vi "DAQ-Hybrid Engine.vi"() -> ()   [LabVIEW 2013]
uses:
  <vilib>/DAQmx/read.llb/DAQmx Read (Analog 1D DBL NChan 1Samp).vi
  <vilib>/Analysis/baseanly.llb/Mean (DBL).vi
  <vilib>/DAQmx/create/channels.llb/DAQmx Create Channel (AI-Voltage-Basic).vi
  <vilib>/DAQmx/configure/timing.llb/DAQmx Timing (Sample Clock).vi
  <vilib>/DAQmx/configure/task.llb/DAQmx Configure Logging (TDMS).vi
  <vilib>/DAQmx/miscellaneous.llb/DAQmx Fill In Error Info.vi
  <resource>/objmgr/daqmx.rc
  <vilib>/Analysis/NI_AALBase.lvlib
panel:
  out "Numeric 2":dbl
  out "Thermometer":dbl(slide) scale=0.0..100.0
  out "Numeric":dbl
  out "Waveform Chart":waveform(dbl)(graph)
  out "?":dbl
  out "Raw":dbl
  in  "File Path 2":path=path "test1.tdms"
  in  "Thrust Offset":dbl format="%0.2f"
  in  "Thrust Slope":dbl=1.0 format="%0.4f"
  in  "Pressure 1 Offset":dbl format="%0.4f"
  in  "Pressure 1 Slope":dbl=1.0 format="%0.2f"
  out "?":dbl
  out "Thrust":dbl(slide) scale=-350.0..350.0
  out "?":dbl
  out "Pressure 1":dbl(knob) scale=0.0..2000.0
  in  "Pressure 1":tag
  in  "?":bool
  in  "?":string="Job 1 - Day 1"
  in  "?":bool
  out "Number of Sensors":sgl
  in  "?":bool
  in  "Samples Per Update":dbl=100.0
  out "Current Group":string="Group 0"
  in  "Sampling Rate [Hz]":i32=10000
  in  "Logging Mode":i32(ring)=15842 items=["Off"=10231, "Log"=15844, "Log and Read"=15842]
  in  "File Path":path=path "test1.tdms"
  # "Data Logging Settings"
  # "Sensor Settings"
  # "Sampling Settings"
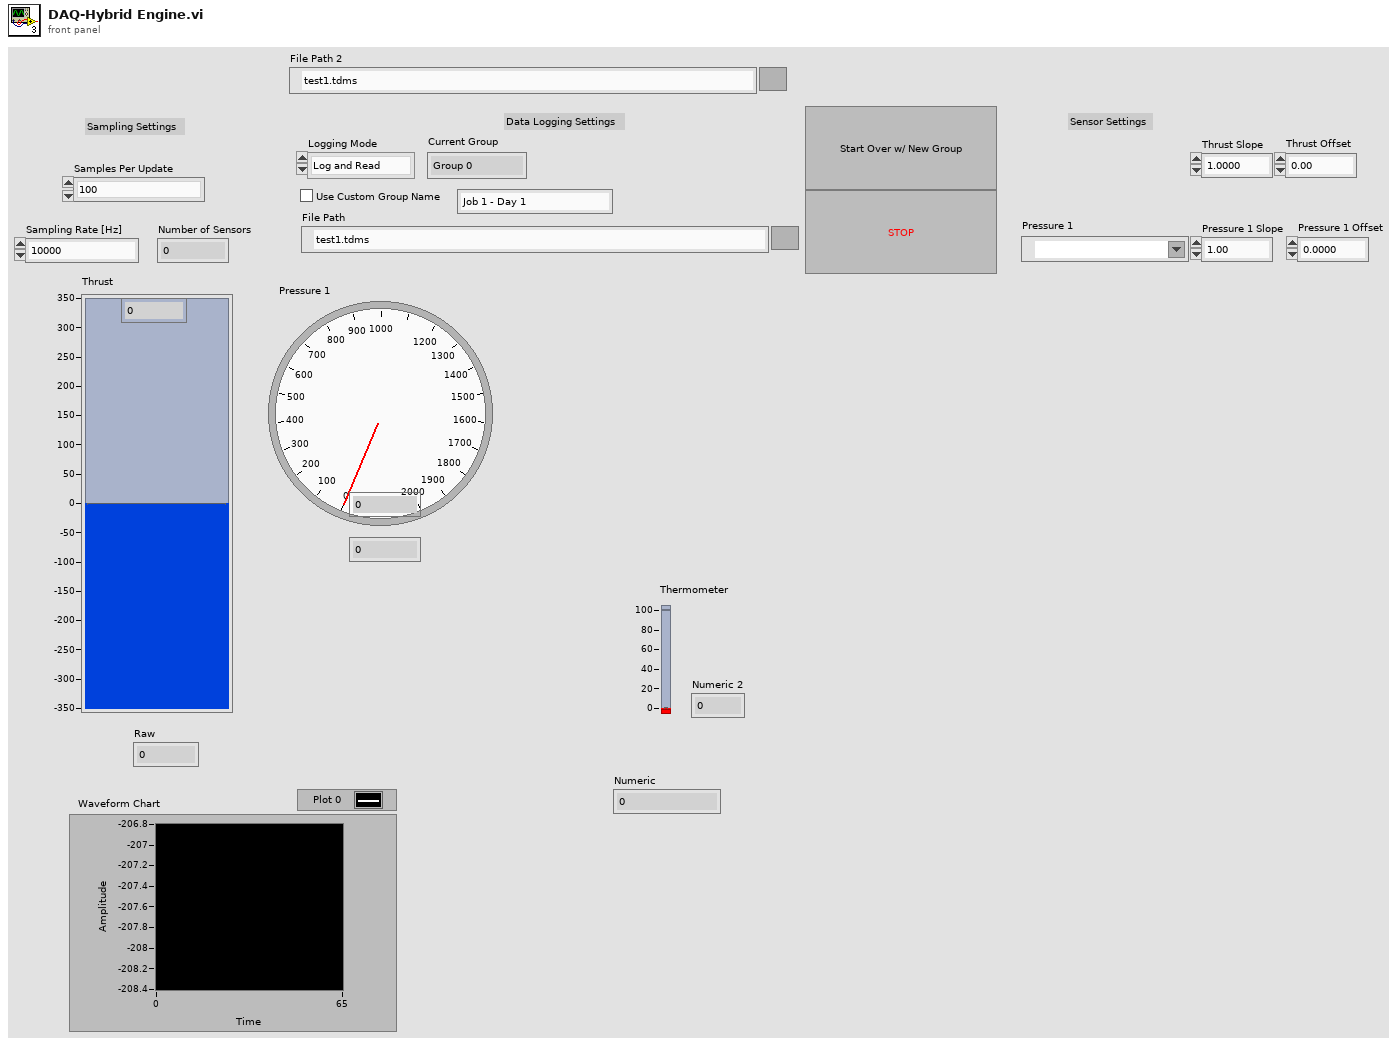
[diagram p1: front panel]
types:
  T1 = enum16{"open", "open or create", "create or replace", "create", "open (read-only)"}
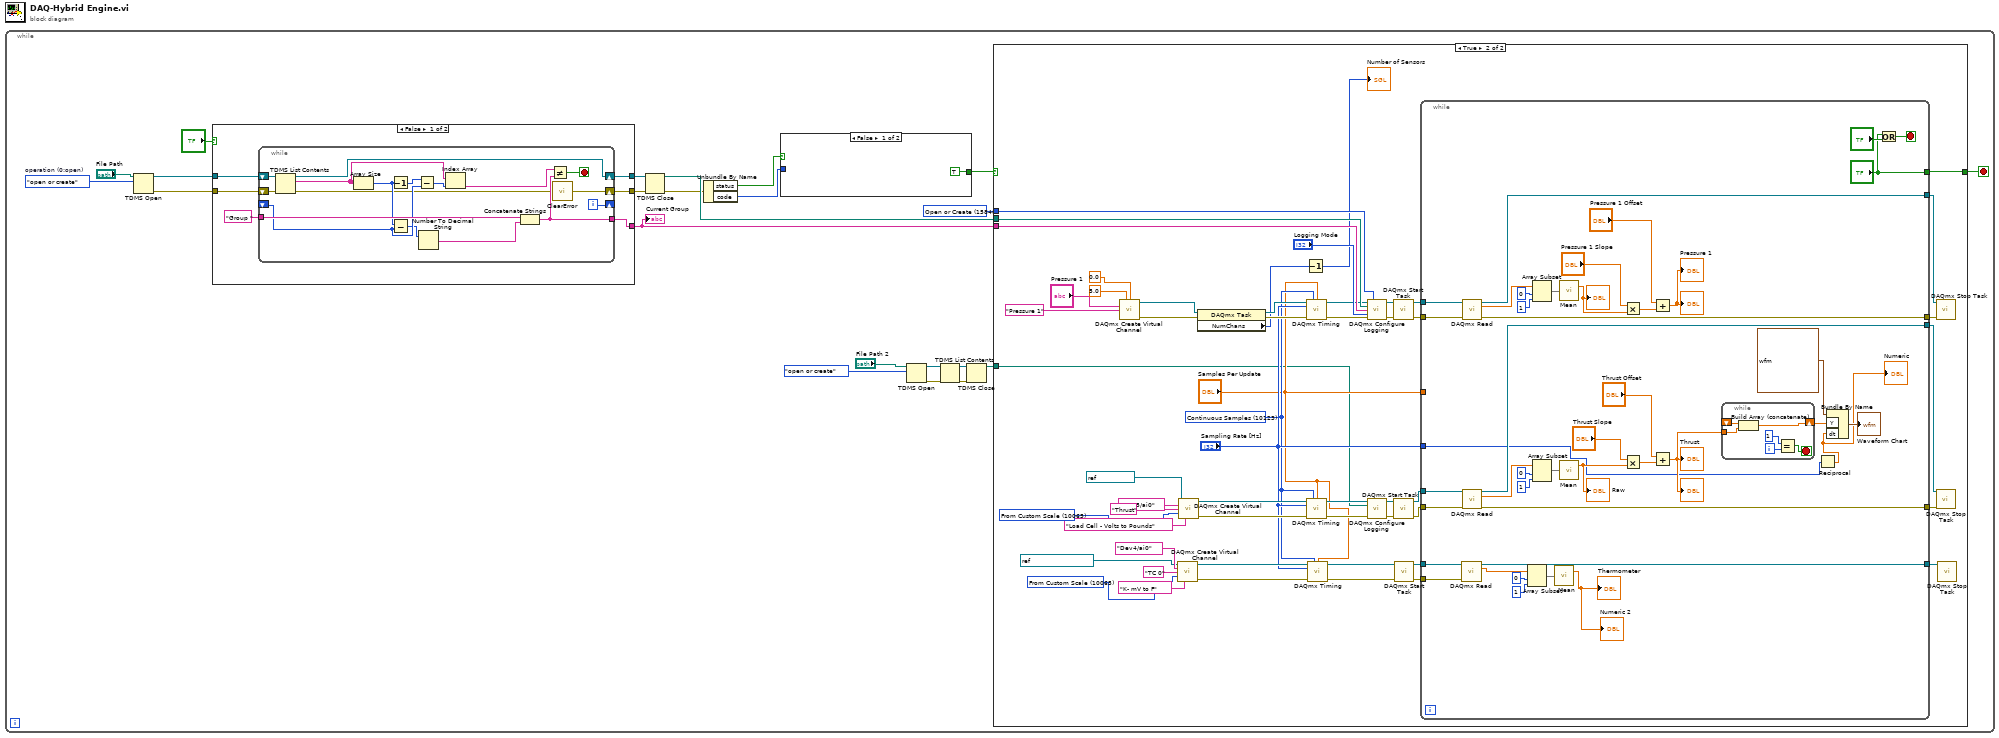
[diagram p0: block diagram]
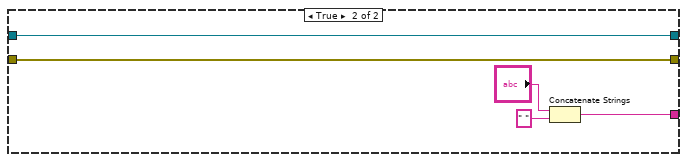
[diagram p2: hidden frame]
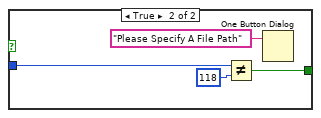
[diagram p3: hidden frame]
diagram:
  n1 = while {
    stop <- w13 stop-if-true
    w19 = T1."open or create"  # operation (0:open)
    w22 = 15846 items=["Open"=10437, "Open or Create"=15846, "Create or Replace"=15847, "Create"=15848] ("operation")
    n2 = TDMS Open(10:w19, 11:"File Path") -> (0:w11:errorcluster, 3:w12:refnum<k34>)  [unwired: 5 in]
    n3 = case shown="False" "?" {
      tunnel: [w25 w48] -> w8
      tunnel: w12 -> [w28 w47]
      tunnel: w11 -> [w27 w46]
      tunnel: [w24 w47] -> w10
      tunnel: [w23 w46] -> w9
      frame False {
        n4 = while {
          shift-right: [w44] -> w24
          shift-left: w28 -> [w45]
          shift-right: [w42] -> w23
          shift-left: w27 -> [w43]
          tunnel: "Group " -> [w40]
          tunnel: [w37] -> w25
          shift-right: [w33] -> _
          shift-left: _ -> [w31]
          i -> [w33]
          stop <- w38 stop-if-true
          n5 = TDMS List Contents(4:w43, 7:w45) -> (0:w29:errorcluster, 2:w36:string[], 3:w44:refnum<k34>)  [unwired: 1 in, 1 out]
          n6 = Array Size(array=w36) -> (size(s)=w32:i32)
          n7 = Decrement(x=w32) -> (x-1=w34:i32)
          n8 = Subtract(x=w32, y=w31) -> (x-y=w30:i32)
          n9 = Subtract(x=w34, y=w31) -> (x-y=w35:i32)
          n10 = Number To Decimal String(number=w30) -> (decimal integer string=w41:string)  [unwired: 1 in]
          n11 = Index Array "Index Array"(array=w36, index=w35) -> (element=w39:string)
          n12 = Concatenate Strings(w40, w41) -> (w37:string)
          n13 = Not Equal?(x=w39, y=w37) -> (x != y?=w38:bool)
          n14 = call <vilib>:"ClearError.vi"("error in (no error)"=w29) -> ("error out"=w42:errorcluster)
        }
      }
      frame True {
        n15 = Concatenate Strings "Concatenate Strings"("?", " ") -> (w48:string)
      }
    }
    "Current Group" <- w8
    n16 = TDMS Close(8:w9, 11:w10) -> (0:w18:errorcluster, 3:w20:path)
    n17 = Unbundle By Name "Unbundle By Name"(w18) -> ("status"=w17:bool, "code"=w16:i32)
    n18 = case shown="False" w17 {
      tunnel: w16 -> [_ w54]
      tunnel: [TRUE w53] -> w15
      frame False {
      }
      frame True {
        n19 = Not Equal?(x=w54, y=118) -> (x != y?=w53:bool)
        n20 = One Button Dialog(message="Please Specify A File Path") -> ()  [unwired: 1 in, 1 out]
      }
    }
    n21 = TDMS Open(10:T1."open or create" ("operation (0:open)"), 11:"File Path 2") -> (0:w4:errorcluster, 3:w5:refnum<k34>)  [unwired: 5 in]
    n22 = TDMS List Contents(4:w4, 7:w5) -> (0:w2:errorcluster, 3:w3:refnum<k34>)  [unwired: 1 in, 2 out]
    n23 = TDMS Close(8:w2, 11:w3) -> (3:w1:path)  [unwired: 1 out]
    n24 = case shown="True" w15 {
      selector: w15 -> [w56 _]
      tunnel: w22 -> [_ w106]
      tunnel: w20 -> [_ w105]
      tunnel: w8 -> [_ w104]
      tunnel: [w56 w95] -> w13
      tunnel: w1 -> [_ w66]
      frame False {
      }
      frame True {
        w65 = 10065 items=["Volts"=10348, "From Custom Scale"=10065] ("units")
        w67 = 10065 items=["Volts"=10348, "From Custom Scale"=10065] ("units")
        w69 = 10123 items=["Finite Samples"=10178, "Continuous Samples"=10123, "Hardware Timed Single Point"=12522] ("sample mode")
        n25 = call-poly <vilib>:"DAQmx Create Virtual Channel.vi"("maximum value"=5.0, "minimum value"=0.0, "physical channels"="Pressure 1", "name to assign"="Pressure 1") -> ("task out"=w87:refnum<k21>, "error out"=w86:errorcluster)  [unwired: 10 in]
        n26 = call-poly <vilib>:"DAQmx Create Virtual Channel.vi"("task in"=refnum<k21> "Thermocouple 0", "physical channels"=tag "Dev4/ai0", "name to assign"="TC 0", "units"=w65, "custom scale name"=tag "K- mV to F") -> ("task out"=w73:refnum<k21>, "error out"=w63:errorcluster)  [unwired: 9 in]
        n27 = call-poly <vilib>:"DAQmx Create Virtual Channel.vi"("task in"=refnum<k21> "Load Cell", "physical channels"=tag "Dev5/ai0", "name to assign"="Thrust", "units"=w67, "custom scale name"=tag "Load Cell - Volts to Pounds") -> ("task out"=w88:refnum<k21>, "error out"=w85:errorcluster)  [unwired: 9 in]
        n28 = property class="DAQmx Task"(reference=w87, error in=w86) -> (reference out=w98:refnum<k21>, error out=w97:errorcluster, "NumChans"=w96:u32)
        n29 = Decrement(x=w96) -> (x-1=→"Number of Sensors":u32)
        n30 = call-poly <vilib>:"DAQmx Timing.vi"("task/channels in"=w98, "sample mode"=w69, "samples per channel"="Samples Per Update", "rate"="Sampling Rate [Hz]", "error in"=w97) -> ("task out"=w99:refnum<k21>, "error out"=w107:errorcluster)  [unwired: 9 in]
        n31 = call-poly <vilib>:"DAQmx Timing.vi"("task/channels in"=w88, "sample mode"=w69, "samples per channel"="Samples Per Update", "rate"="Sampling Rate [Hz]", "error in"=w85) -> ("task out"=w82:refnum<k21>, "error out"=w81:errorcluster)  [unwired: 9 in]
        n32 = call-poly <vilib>:"DAQmx Timing.vi"("task/channels in"=w73, "sample mode"=w69, "samples per channel"="Samples Per Update", "rate"="Sampling Rate [Hz]", "error in"=w63) -> ("task out"=w64:refnum<k21>, "error out"=w62:errorcluster)  [unwired: 9 in]
        n33 = call-poly <vilib>:"DAQmx Configure Logging.vi"("task/channels in"=w99, "operation"=w106, "file path"=w105, "group name"=w104, "logging mode"="Logging Mode", "error in"=w107) -> ("task out"=w110:refnum<k21>, "error out"=w109:errorcluster)  [unwired: 8 in]
        n34 = call-poly <vilib>:"DAQmx Configure Logging.vi"("task/channels in"=w82, "file path"=w66, "error in"=w81) -> ("task out"=w84:refnum<k21>, "error out"=w83:errorcluster)  [unwired: 11 in]
        n35 = call <vilib>:"DAQmx Start Task.vi"("task/channels in"=w110, "error in"=w109) -> ("task out"=w103:refnum<k21>, "error out"=w102:errorcluster)  [unwired: 12 in]
        n36 = call <vilib>:"DAQmx Start Task.vi"("task/channels in"=w84, "error in"=w83) -> ("task out"=w80:refnum<k21>, "error out"=w79:errorcluster)  [unwired: 12 in]
        n37 = call <vilib>:"DAQmx Start Task.vi"("task/channels in"=w64, "error in"=w62) -> ("task out"=w72:refnum<k21>, "error out"=w61:errorcluster)  [unwired: 12 in]
        n38 = while {
          tunnel: w103 -> [w152]
          tunnel: w102 -> [w151]
          tunnel: [w150] -> w101
          tunnel: [w149] -> w100
          tunnel: ["?"] -> w95
          tunnel: w80 -> [w139]
          tunnel: w79 -> [w138]
          tunnel: [w121] -> w78
          tunnel: [w136] -> w77
          tunnel: "Sampling Rate [Hz]" -> [w120]
          tunnel: "Samples Per Update" -> [_]
          tunnel: w72 -> [w118]
          tunnel: [w117] -> w71
          tunnel: w61 -> [w116]
          stop <- w140 stop-if-true
          n39 = call-poly <vilib>:"DAQmx Read.vi"("task/channels in"=w118, "error in"=w116) -> ("task out"=w117:refnum<k21>, "data"=w112:dbl[])  [unwired: 11 in, 1 out]
          n40 = call-poly <vilib>:"DAQmx Read.vi"("task/channels in"=w152, "error in"=w151) -> ("task out"=w150:refnum<k21>, "data"=w144:dbl[], "error out"=w149:errorcluster)  [unwired: 11 in]
          n41 = call-poly <vilib>:"DAQmx Read.vi"("task/channels in"=w139, "error in"=w138) -> ("task out"=w121:refnum<k21>, "data"=w137:dbl[], "error out"=w136:errorcluster)  [unwired: 11 in]
          n42 = Array Subset(array=w112, index=0, length=1) -> (w115:dbl[])
          n43 = Array Subset(array=w144, index=0, length=1) -> (w141:dbl[])
          n44 = Array Subset(array=w137, index=0, length=1) -> (w135:dbl[])
          n45 = call-poly <vilib>:"Mean.vi"("X"=w115) -> ("mean"=→"Thermometer" →"Numeric 2":dbl)  [unwired: 1 out]
          n46 = call-poly <vilib>:"Mean.vi"("X"=w141) -> ("mean"=w126:dbl)  [unwired: 1 out]
          "?" <- w126
          n47 = call-poly <vilib>:"Mean.vi"("X"=w135) -> ("mean"=w131:dbl)  [unwired: 1 out]
          "Raw" <- w131
          n48 = Multiply(x="Pressure 1 Slope", y=w126) -> (x*y=w130:dbl)
          n49 = Multiply(x="Thrust Slope", y=w131) -> (x*y=w134:dbl)
          n50 = Add(x="Pressure 1 Offset", y=w130) -> (x+y=→"Pressure 1" →"?":dbl)
          n51 = Add(x="Thrust Offset", y=w134) -> (x+y=w125:dbl)
          "Thrust" <- w125
          "?" <- w125
          n52 = while {
            tunnel: w125 -> [w158]
            shift-right: [w157] -> w122
            shift-left: _ -> [w156]
            i -> [w155]
            stop <- w154 stop-if-true
            n53 = Build Array (concatenate)(w156, w158) -> (w157:dbl[])
            n54 = Equal?(x=1, y=w155) -> (x = y?=w154:bool)
          }
          n55 = Reciprocal(x=w120) -> (1/x=w119:dbl)
          "Numeric" <- w119
          n56 = Bundle By Name(cluster=waveform(dbl) {"t0"=timestamp(0 s since 1904-01-01), "dt"=1.0, "Y"=[]} ("waveform"), "Y"=w122, "dt"=w119) -> (→"Waveform Chart":waveform(dbl))
          n57 = Or(x="?", y="?") -> (x .or. y?=w140:bool)
        }
        n58 = call <vilib>:"DAQmx Stop Task.vi"("task/channels in"=w101, "error in"=w100) -> ()  [unwired: 12 in, 2 out]
        n59 = call <vilib>:"DAQmx Stop Task.vi"("task/channels in"=w78, "error in"=w77) -> ()  [unwired: 12 in, 2 out]
        n60 = call <vilib>:"DAQmx Stop Task.vi"("task/channels in"=w71) -> ()  [unwired: 13 in, 2 out]
      }
    }
  }
